vi "Start Build.vi"(0 "Open Directory?":bool, 1 "Build Packge?":bool, 2 "Progres Bar":refnum<vi>, 5 "Feed":T2(ring), 7 "Feed Path":path, 9 "Selected Meas":T1[](array[typedef]), 11 "error in (no error)":errorcluster, 12 "Package Spec":string[][](array[string])) -> (4 "Status":string[](array[string]), 15 "error out":errorcluster)   [LabVIEW 2021, in "Measurement Builder.lvlib"]
uses:
  Measurement Builder.lvlib
  controls/Build Spec Details.ctl
  <vilib>/AppBuilder/AB_API_Simple/Set Build Specification Version (path).vi
  <vilib>/AppBuilder/AB_API_Simple/Build (path).vi
  Dictionary/Dictionary.lvlib
  <vilib>/AppBuilder/AB_API_Simple/NI_App_Builder_API.lvlib
  Path Functions/Path Functions.lvlib
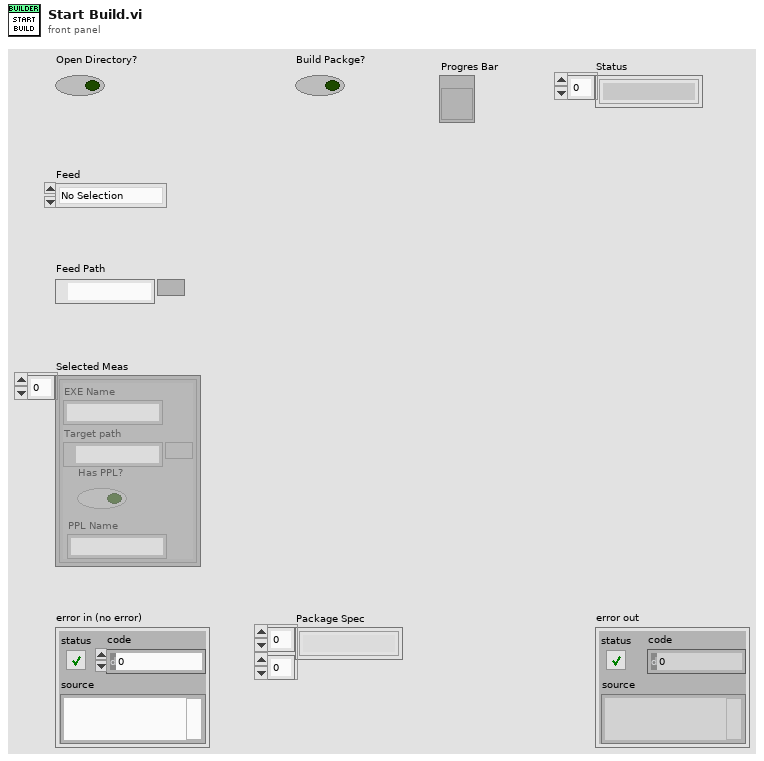
[diagram p1: front panel]
types:
  T1 = typedef "Measurement Builder.lvlib/Build Spec Details.ctl" = cluster{"EXE Name":string, "Target path":path, "Has PPL?":bool, "PPL Name":string}
  T2 = enum32{"No Selection", "CreateFeed", "AddtoFeed"}
  T3 = typedef "NI_App_Builder_API.lvlib/Build Specification Version.ctl" = cluster{"Major":u16, "Minor":u16, "Fix":u16, "Build":u16}
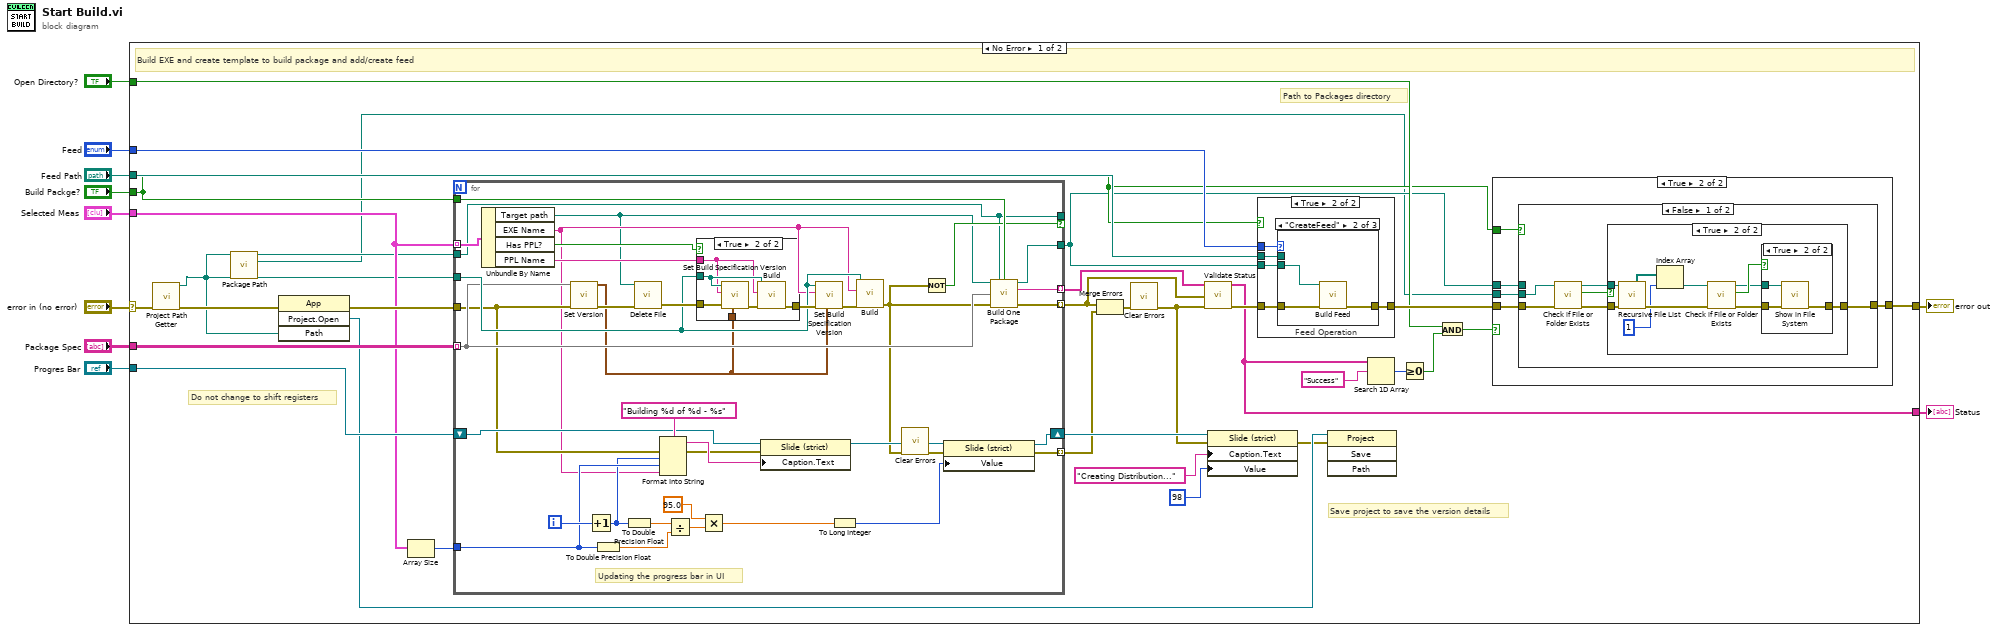
[diagram p0: block diagram]
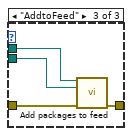
[diagram p4: hidden frame]
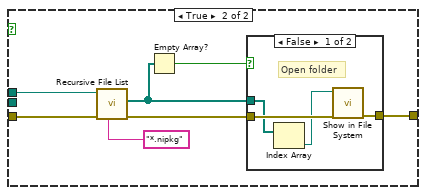
[diagram p9: hidden frame]
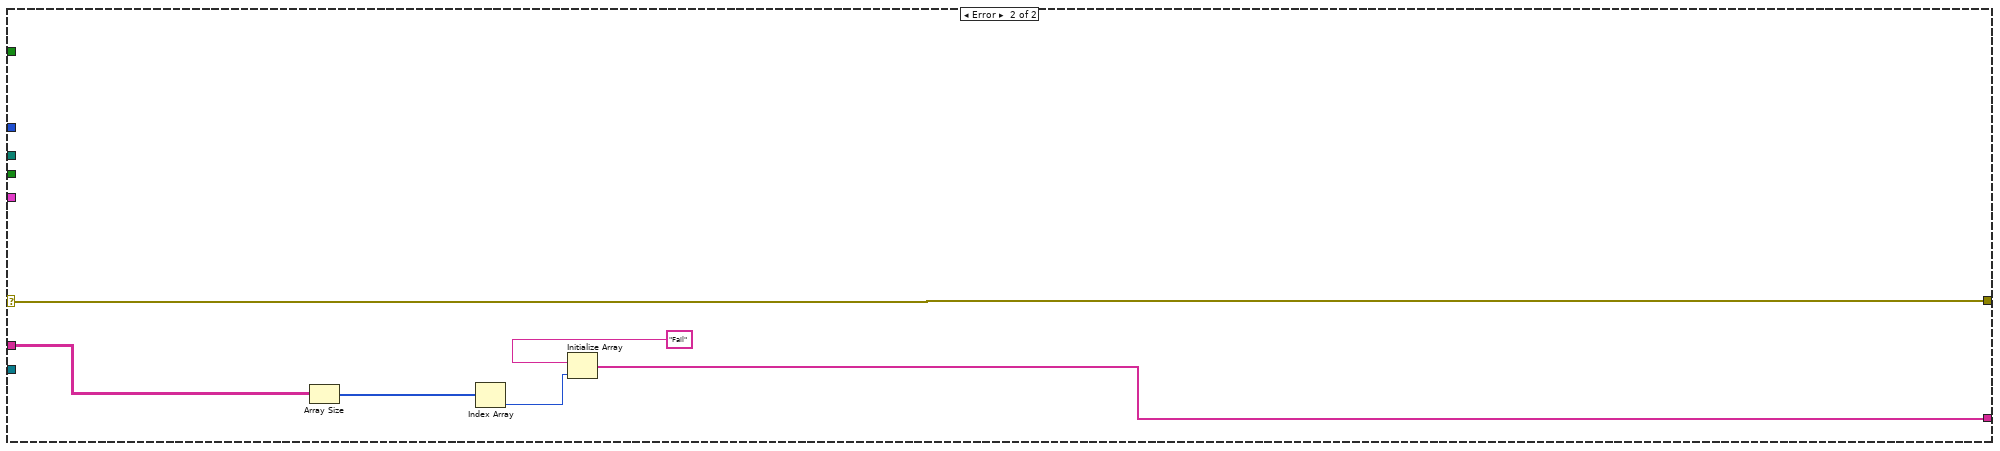
[diagram p11: hidden frame]
diagram:
  n1 = case shown="No Error" "error in (no error)" {
    selector: "error in (no error)" -> [w30 w146]
    tunnel: "Package Spec" -> [w43 w144]
    tunnel: [w34 w146] -> w8
    tunnel: [w21 w141] -> w7
    tunnel: "Progres Bar" -> [w40 _]
    tunnel: "Open Directory?" -> [w16 _]
    tunnel: "Feed" -> [w24 _]
    tunnel: "Feed Path" -> [w23 _]
    tunnel: "Build Packge?" -> [w13 _]
    tunnel: "Selected Meas" -> [w22 _]
    frame No Error {
      # "Path to Packages directory"
      # "Save project to save the version details"
      # "Do not change to shift registers"
      # "Build EXE and create template to build package and add/create feed"
      n2 = call "Project Path Getter.vi"("error in (no error)"=w30) -> ("Path"=w14:path, "error out"=w29:errorcluster)  [unwired: 13 in]
      n3 = call "Package Path.vi"("Path"=w14) -> ("Package Path"=w15:path, "Build Outputs"=w11:path)  [unwired: 13 in]
      n4 = invoke class="App" method="Project.Open"(error in=w29, "Path"=w14) -> (error out=w31:errorcluster, "Project:Open"=w28:refnum<vi>)  [unwired: 2 in, 2 out]
      n5 = Array Size(array=w22) -> (size(s)=w39:i32)
      n6 = for {
        tunnel: w31 -> [w65]
        tunnel: w22 -> [w94] mode=indexing
        tunnel: w13 -> [w80]
        tunnel: w43 -> [w66] mode=indexing
        tunnel: [w93] -> w12
        tunnel: [w92] -> w42 mode=indexing
        tunnel: [w91] -> w41 mode=indexing
        tunnel: w39 -> [w86]
        tunnel: [w76] -> w32 mode=indexing
        shift-right: [w73] -> w35
        shift-left: w40 -> [w88]
        tunnel: [w58] -> _ if=w60
        tunnel: w14 -> [w67]
        tunnel: w15 -> [w58]
        i -> [w89]
        # "Updating the progress bar in UI"
        n7 = Unbundle By Name(w94) -> ("Target path"=w59:path, "EXE Name"=w63:string, "Has PPL?"=w70:bool, "PPL Name"=w69:string)
        n8 = call "Set Version.vi"("Package Spec"=w66, "error in (no error)"=w65) -> ("Build Specification Version"=w62:T3, "error out"=w64:errorcluster)  [unwired: 12 in]
        n9 = Increment(x=w89) -> (x+1=w85:i32)
        n10 = To Double Precision Float(number=w86) -> (double precision float=w79:dbl)
        n11 = To Double Precision Float(number=w85) -> (double precision float=w81:dbl)
        n12 = call "Delete File.vi"("Path"=w59, "error in (no error)"=w64) -> ("error out"=w71:errorcluster)  [unwired: 13 in]
        n13 = Format Into String(format string="Building %d of %d - %s", error in=w65, w85, w86, w63) -> (resulting string=w87:string, error out=w78:errorcluster)  [unwired: 1 in]
        n14 = Divide(x=w81, y=w79) -> (x/y=w84:dbl)
        n15 = case shown="True" w70 {
          tunnel: w67 -> [_ w100]
          tunnel: [w95 w96] -> w72
          tunnel: w71 -> [w95 w101]
          tunnel: w69 -> [_ w99]
          tunnel: w62 -> [_ w98]
          frame False {
          }
          frame True {
            n16 = call-poly <vilib>:"Set Build Specification Version.vi"("Build Specification Version"=w98, "error in (no error)"=w101, "Name of build specification"=w99, "Path to project"=w100) -> ("error out"=w97:errorcluster)  [unwired: 7 in]
            n17 = call-poly <vilib>:"Build.vi"("error in (no error)"=w97, "Name of build specification (if empty: build all)"=w99, "Path to project"=w100) -> ("error out"=w96:errorcluster)  [unwired: 7 in, 1 out]
          }
        }
        n18 = Multiply(x=95.0 ("y"), y=w84) -> (x*y=w82:dbl)
        n19 = property class="Slide (strict)"(reference=w88, error in=w78, "Caption.Text"=w87) -> (reference out=w74:refnum<vi>)  [unwired: 1 out]
        n20 = call-poly <vilib>:"Set Build Specification Version.vi"("Build Specification Version"=w62, "error in (no error)"=w72, "Name of build specification"=w63, "Path to project"=w67) -> ("error out"=w68:errorcluster)  [unwired: 7 in]
        n21 = To Long Integer(number=w82) -> (32bit integer=w75:i32)
        n22 = call-poly <vilib>:"Build.vi"("error in (no error)"=w68, "Name of build specification (if empty: build all)"=w63, "Path to project"=w67) -> ("error out"=w61:errorcluster)  [unwired: 7 in, 1 out]
        n23 = call <vilib>:"Clear Errors.vi"("error in (no error)"=w61) -> ("error out"=w77:errorcluster)  [unwired: 5 in, 1 out]
        n24 = Not(x=w61) -> (.not. x?=w60:bool)
        n25 = property class="Slide (strict)"(reference=w74, error in=w77, "Value"=w75) -> (reference out=w73:refnum<vi>, error out=w76:errorcluster)
        n26 = call "Build One Package.vi"("Destination Path"=w59, "Package Path"=w58, "Build Packge?"=w80, "Package Spec"=w66, "error in (no error)"=w61) -> ("Package Directory"=w93:path, "Error Message"=w91:string, "error out"=w92:errorcluster)  [unwired: 8 in]
      }
      n27 = Merge Errors(w42, w32) -> (w38:errorcluster)
      n28 = call <vilib>:"Clear Errors.vi"("error in (no error)"=w38) -> ("error out"=w25:errorcluster)  [unwired: 5 in, 1 out]
      n29 = call "Validate Status.vi"("Error Msg[]"=w41, "Error[]"=w42, "error in (no error)"=w25) -> ("Status"=w21:string[], "error out"=w26:errorcluster)  [unwired: 11 in]
      n30 = property class="Slide (strict)"(reference=w35, error in=w25, "Caption.Text"="Creating Distribution...", "Value"=98) -> (error out=w27:errorcluster)  [unwired: 1 out]
      n31 = case shown="True" w13 {
        tunnel: w24 -> [_ w49]
        tunnel: w23 -> [_ w48]
        tunnel: w26 -> [w44 w47]
        tunnel: [w44 w46] -> w33
        tunnel: w12 -> [_ w45]
        frame False {
        }
        frame True {
          n32 = case "Feed Operation" shown="\"CreateFeed\"" w49 {
            tunnel: w47 -> [w50 w51 w54]
            tunnel: w48 -> [_ _ w57]
            tunnel: [w50 w53 w55] -> w46
            tunnel: w45 -> [_ w52 w56]
            frame "No Selection" {
            }
            frame "CreateFeed" {
              n33 = call "Build Feed.vi"("Packages Path"=w52, "error in (no error)"=w51) -> ("error out"=w53:errorcluster)  [unwired: 13 in]
            }
            frame "AddtoFeed" {
              n34 = call "Add packages to feed.vi"("Feed Path"=w57, "Packages Path"=w56, "error in (no error)"=w54) -> ("error out"=w55:errorcluster)  [unwired: 12 in]
            }
          }
        }
      }
      n35 = invoke class="Project" method="Save"(reference=w28, error in=w27) -> ()  [unwired: 2 in, 4 out]
      n36 = Search 1D Array(1D array=w21, element="Success") -> (index of element=w19:i32)  [unwired: 1 in]
      n37 = Greater Or Equal To 0?(x=w19) -> (x >= 0?=w18:bool)
      n38 = And(x=w16, y=w18) -> (x .and. y?=w17:bool)
      n39 = case shown="True" w17 {
        tunnel: w33 -> [w102 w106]
        tunnel: [w102 w107] -> w34
        tunnel: w13 -> [_ w105]
        tunnel: w12 -> [_ w104]
        tunnel: w11 -> [_ w103]
        frame False {
        }
        frame True {
          n40 = case shown="False" w105 {
            tunnel: [w113 w135] -> w107
            tunnel: w106 -> [w112 w133]
            tunnel: w104 -> [_ w129]
            tunnel: w103 -> [w108 _]
            frame False {
              n41 = call <vilib>:"Check if File or Folder Exists.vi"("error in (no error)"=w112, "path"=w108) -> ("error out"=w111:errorcluster, "file or folder exists?"=w109:bool, "dup path"=w110:path)  [unwired: 7 in]
              n42 = case shown="True" w109 {
                tunnel: [w114 w124] -> w113
                tunnel: w111 -> [w114 w117]
                tunnel: w110 -> [_ w116]
                frame False {
                }
                frame True {
                  n43 = call <vilib>:"Recursive File List.vi"("error in (no error)"=w117, "Folder Path"=w116) -> ("error out"=w119:errorcluster, "All Folders"=w123:path[])  [unwired: 5 in, 3 out]
                  n44 = Index Array(array=w123, index=1) -> (element=w122:path)
                  n45 = call <vilib>:"Check if File or Folder Exists.vi"("error in (no error)"=w119, "path"=w122) -> ("error out"=w120:errorcluster, "file or folder exists?"=w121:bool, "dup path"=w118:path)  [unwired: 7 in]
                  n46 = case shown="True" w121 {
                    tunnel: [w125 w128] -> w124
                    tunnel: w120 -> [w125 w127]
                    tunnel: w118 -> [_ w126]
                    frame False {
                    }
                    frame True {
                      n47 = call <vilib>:"Show in File System.vi"("error in (no error)"=w127, "file or directory path"=w126) -> ("error out"=w128:errorcluster)  [unwired: 9 in]
                    }
                  }
                }
              }
            }
            frame True {
              n48 = call <vilib>:"Recursive File List.vi"("pattern"="*.nipkg", "error in (no error)"=w133, "Folder Path"=w129) -> ("error out"=w132:errorcluster, "All Files in Dir"=w131:path[])  [unwired: 4 in, 3 out]
              n49 = Empty Array?(array=w131) -> (empty?=w130:bool)
              n50 = case shown="False" w130 {
                tunnel: [w139 w140] -> w135
                tunnel: w132 -> [w138 w140]
                tunnel: w131 -> [w137 _]
                frame False {
                  # "Open folder"
                  n51 = Index Array(array=w137) -> (element=w136:path)  [unwired: 1 in]
                  n52 = call <vilib>:"Show in File System.vi"("error in (no error)"=w138, "file or directory path"=w136) -> ("error out"=w139:errorcluster)  [unwired: 9 in]
                }
                frame True {
                }
              }
            }
          }
        }
      }
    }
    frame Error {
      n53 = Array Size(array=w144) -> (size(s)=w143:i32[])
      n54 = Index Array(array=w143) -> (element=w142:i32)  [unwired: 1 in]
      n55 = Initialize Array("Fail", w142) -> (w141:string[])
    }
  }
  "error out" <- w8
  "Status" <- w7
